vi "connection_process.vi"(6 "timeout (ms)":i32=1000, 11 "Connection":refnum<class "Connection.lvclass">) -> ()   [LabVIEW 2013, in "MQTT_Connection.lvlib" / "Connection.lvclass"]
uses:
  Connection.lvclass
  Connection.lvclass/Connection.ctl
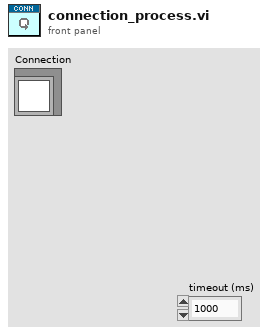
[diagram p1: front panel]
types:
  T1 = cluster{"Connection":refnum<class "Connection.lvclass">, "error out":errorcluster}
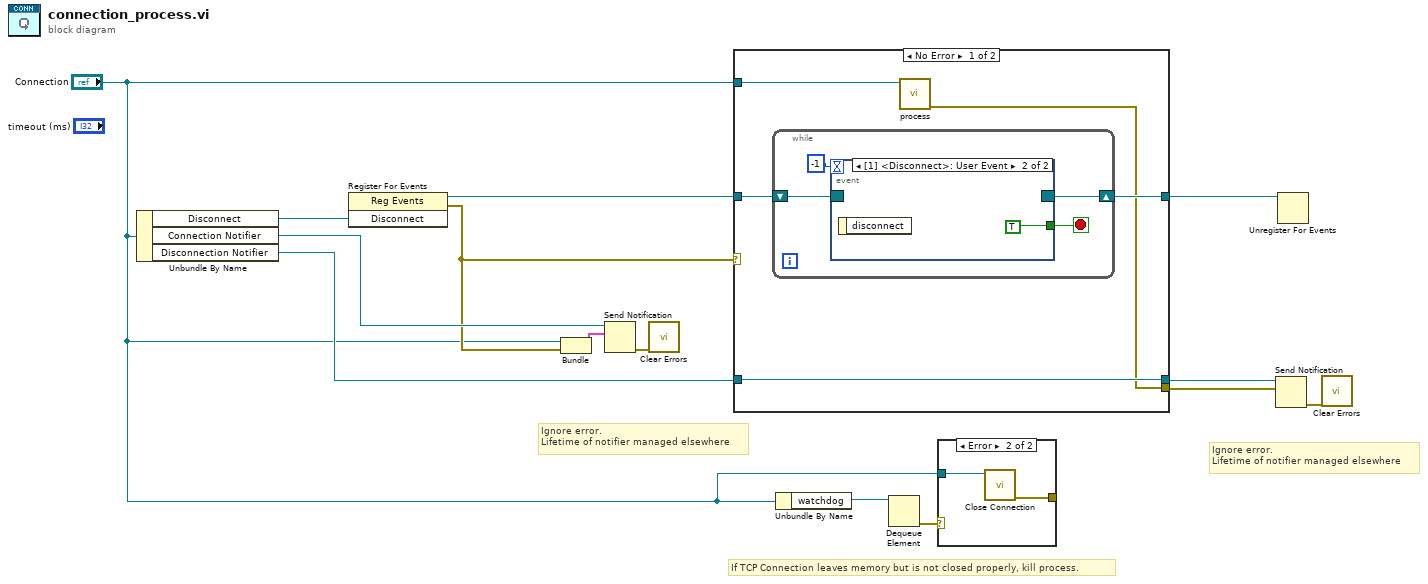
[diagram p0: block diagram]
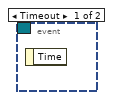
[diagram p3: hidden frame]
diagram:
  # "If TCP Connection leaves memory but is not closed properly, kill process."
  # "Ignore error.\nLifetime of notifier managed elsewhere"
  # "Ignore error.\nLifetime of notifier managed elsewhere"
  n1 = Unbundle By Name("Connection") -> ("Disconnect"=w11:refnum<user-event>, "Connection Notifier"=w10:refnum<notifier>, "Disconnection Notifier"=w6:refnum<notifier>)
  n2 = register-events(w11) -> (reference out=w12:refnum<event-registration>, error out=w3:errorcluster)  [unwired: 2 in]
  n3 = Bundle("Connection"="Connection", "error out"=w3) -> (w14:T1)  [unwired: 1 in]
  n4 = Send Notification(notification=w14, notifier=w10) -> (error out=w1:errorcluster)  [unwired: 1 in, 1 out]
  n5 = call <vilib>:"Clear Errors.vi"("error in (no error)"=w1) -> ()  [unwired: 6 in, 1 out]
  n6 = case shown="No Error" w3 {
    selector: w3 -> [_ w26]
    tunnel: [w19 w27] -> w13
    tunnel: w12 -> [w18 w27]
    tunnel: [w15 w26] -> w9
    tunnel: w6 -> [w17 w25]
    tunnel: [w17 w25] -> w8
    tunnel: "Connection" -> [w16 _]
    frame No Error {
      n7 = while {
        shift-right: [w22] -> w19
        shift-left: w18 -> [w21]
        stop <- w20 stop-if-true
        n8 = event shown="[1] <Disconnect>: User Event" {
          selector: w21 -> [_ _]
          dyn-events: [_ _] -> w22
          timeout: -1 -> [_ _]
          tunnel: [_ TRUE] -> w20
          event Timeout {
            n9 = event-data() -> ()  [unwired: 1 in, 1 out]
          }
          event User Event {
            n10 = event-data() -> ()  [unwired: 1 in, 1 out]
          }
        }
      }
      n11 = call-dynamic "process.vi"("Connection in"=w16) -> ("error out"=w15:errorcluster)  [unwired: 9 in, 1 out]
    }
    frame Error {
    }
  }
  n12 = Unbundle By Name("Connection") -> ("watchdog"=w5:refnum<queue>)
  n13 = Dequeue Element(queue=w5) -> (error out=w4:errorcluster)  [unwired: 2 in, 3 out]
  n14 = case shown="Error" w4 {
    tunnel: [_ w28] -> _
    tunnel: "Connection" -> [_ w29]
    frame No Error {
    }
    frame Error {
      n15 = call-dynamic "Close Connection.vi"("Connection in"=w29) -> ("error out"=w28:errorcluster)  [unwired: 9 in, 1 out]
    }
  }
  n16 = Send Notification(notification=w9, notifier=w8) -> (error out=w7:errorcluster)  [unwired: 1 in, 1 out]
  n17 = Unregister For Events(event registration refnum=w13) -> ()  [unwired: 1 in, 1 out]
  n18 = call <vilib>:"Clear Errors.vi"("error in (no error)"=w7) -> ()  [unwired: 6 in, 1 out]
